vi "Excel_Get_Range.vi"(0 "Excel._Worksheet":refnum<k7>, 5 "start":cluster{"row":i32, "column":i32}={"row"=-1, "column"=-1}, 7 "end":cluster{"row":i32, "column":i32}={"row"=-1, "column"=-1}, 9 "name":string, 11 "error in (no error)":errorcluster) -> (4 "Range":refnum<k7>, 15 "error out":errorcluster)   [LabVIEW 2020, in "NI_ReportGenerationToolkit.lvlib"]
uses:
  <vilib>/addons/_office/NI_ReportGenerationToolkit.lvlib
  <vilib>/Utility/NIReport.llb/NI_ReportGenerationCore.lvlib
panel:
  in  "Excel.Range":refnum<k7>
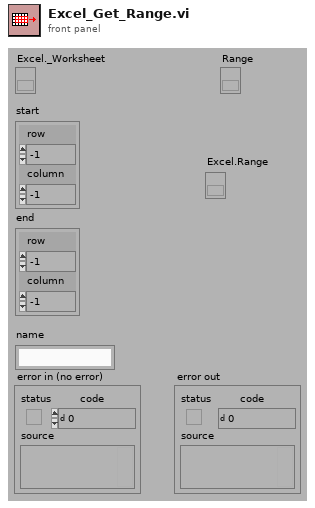
[diagram p1: front panel]
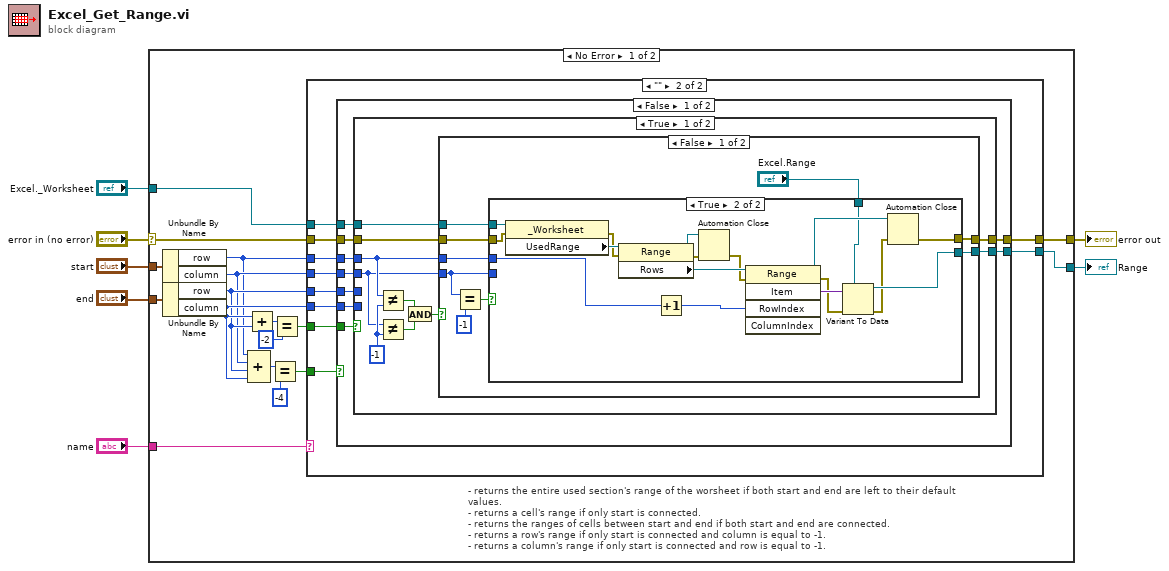
[diagram p0: block diagram]
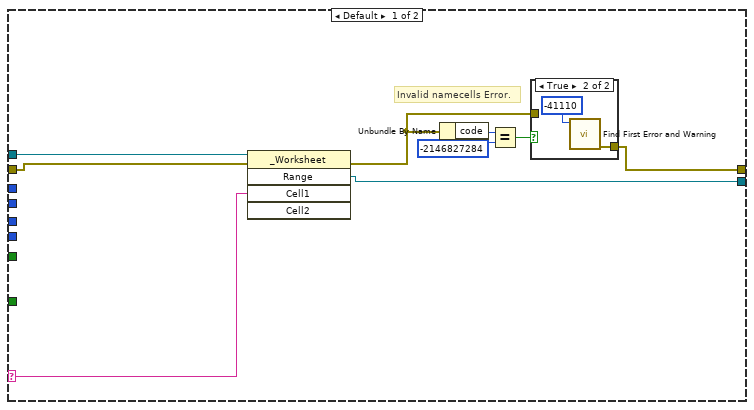
[diagram p2: hidden frame]
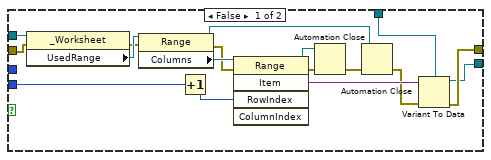
[diagram p4: hidden frame]
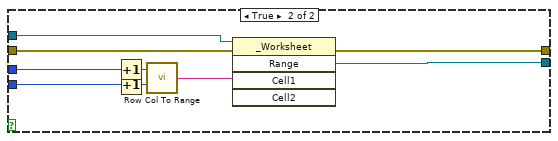
[diagram p5: hidden frame]
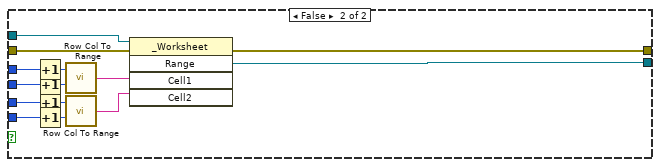
[diagram p6: hidden frame]
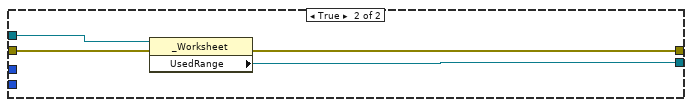
[diagram p7: hidden frame]
diagram:
  n1 = case shown="No Error" "error in (no error)" {
    selector: "error in (no error)" -> [w8 w136]
    tunnel: [w24 _] -> w7
    tunnel: "end" -> [w13 _]
    tunnel: "start" -> [w12 _]
    tunnel: "Excel._Worksheet" -> [w11 _]
    tunnel: [w10 w136] -> w3
    tunnel: "name" -> [w9 _]
    frame No Error {
      # "- returns the entire used section's range of the worsheet if both start and end are left to their default values.\n- returns a cell's range if only start is connected.\n- returns the ranges of cells between start and end if both start and end are connected.\n- returns a row's range if only start is connected and column is equal to -1.\n- returns a column's range if only start is connected and row is equal to -1."
      n2 = Unbundle By Name(w12) -> ("row"=w18:i32, "column"=w19:i32)
      n3 = Unbundle By Name(w13) -> ("row"=w20:i32, "column"=w21:i32)
      n4 = Add(x=w21, y=w20) -> (x+y=w17:i32)
      n5 = Compound Arithmetic op=ADD(w18, w19, w20, w21) -> (w14:i32)
      n6 = Equal?(x=w14, y=-4) -> (x = y?=w23:bool)
      n7 = Equal?(x=w17, y=-2) -> (x = y?=w22:bool)
      n8 = case shown="\"\"" w9 {
        selector: w9 -> [w25 _]
        tunnel: [w31 w46] -> w24
        tunnel: w8 -> [w32 w45]
        tunnel: w23 -> [_ w44]
        tunnel: w22 -> [_ w43]
        tunnel: w21 -> [_ w42]
        tunnel: w20 -> [_ w41]
        tunnel: w19 -> [_ w40]
        tunnel: w18 -> [_ w39]
        tunnel: w11 -> [w33 w38]
        tunnel: [w26 w37] -> w10
        frame Default {
          # "Invalid namecells Error."
          n9 = invoke on="Invoke Node" class="_Worksheet" method="Range"(reference=w33, error in=w32, "Cell1"=w25) -> (error out=w27:errorcluster, "Range"=w31:refnum<k7>)  [unwired: 2 in, 3 out]
          n10 = Unbundle By Name(w27) -> ("code"=w29:i32)
          n11 = Equal?(x=w29, y=-2146827284) -> (x = y?=w30:bool)
          n12 = case shown="True" w30 {
            tunnel: [w34 w35] -> w26
            tunnel: w27 -> [w34 _]
            frame False {
            }
            frame True {
              n13 = call <vilib>:"Find First Error and Warning.vi"("error code"=-41110) -> ("error out"=w35:errorcluster)  [unwired: 1 in, 5 out]
            }
          }
        }
        frame "" {
          n14 = case shown="False" w44 {
            tunnel: w38 -> [w54 w133]
            tunnel: w45 -> [w51 w132]
            tunnel: [w49 w135] -> w46
            tunnel: [w50 w134] -> w37
            tunnel: w43 -> [w55 _]
            tunnel: w39 -> [w53 _]
            tunnel: w40 -> [w52 _]
            tunnel: w41 -> [w48 _]
            tunnel: w42 -> [w47 _]
            frame False {
              n15 = case shown="True" w55 {
                tunnel: w54 -> [w65 w131]
                tunnel: w53 -> [w60 w130]
                tunnel: w52 -> [w59 w129]
                tunnel: w51 -> [w64 w125]
                tunnel: [w63 w124] -> w50
                tunnel: [w62 w123] -> w49
                tunnel: w48 -> [_ w120]
                tunnel: w47 -> [_ w119]
                frame True {
                  w61 = -1
                  n16 = Not Equal?(x=w60, y=w61) -> (x != y?=w57:bool)
                  n17 = Not Equal?(x=w59, y=w61) -> (x != y?=w56:bool)
                  n18 = And(x=w57, y=w56) -> (x .and. y?=w58:bool)
                  n19 = case shown="False" w58 {
                    tunnel: w65 -> [w70 w117]
                    tunnel: w60 -> [w74 w116]
                    tunnel: w59 -> [w73 w115]
                    tunnel: w64 -> [w69 w112]
                    tunnel: [w67 w111] -> w63
                    tunnel: [w68 w110] -> w62
                    frame False {
                      n20 = Equal?(x=w73, y=-1) -> (x = y?=w71:bool)
                      n21 = case shown="True" w71 {
                        tunnel: w73 -> [w90 _]
                        tunnel: w74 -> [_ w107]
                        tunnel: w70 -> [w82 w99]
                        tunnel: w69 -> [w80 w98]
                        tunnel: "Excel.Range" -> [w75 w92]
                        tunnel: [w84 w104] -> w68
                        tunnel: [w85 w102] -> w67
                        frame False {
                          n22 = property on="Property Node" class="_Worksheet"(reference=w82, error in=w80) -> (error out=w79:errorcluster, "UsedRange"=w81:refnum<k7>)  [unwired: 1 out]
                          n23 = property on="Property Node" class="Range"(reference=w81, error in=w79) -> (reference out=w76:refnum<k7>, error out=w87:errorcluster, "Columns"=w91:refnum<k7>)
                          n24 = Increment(x=w90) -> (x+1=w89:i32)
                          n25 = invoke on="Invoke Node" class="Range" method="Item"(reference=w91, error in=w87, "RowIndex"=w89) -> (reference out=w83:refnum<k7>, error out=w88:errorcluster, "Item"=w86:variant)  [unwired: 2 in, 2 out]
                          n26 = Automation Close(3:w88, 5:w83) -> (0:w78:errorcluster)
                          n27 = Automation Close(3:w78, 5:w76) -> (0:w77:errorcluster)
                          n28 = Variant To Data(error in=w77, type=w75, Variant=w86) -> (data=w84:refnum<k7>, error out=w85:errorcluster)
                        }
                        frame True {
                          n29 = property on="Property Node" class="_Worksheet"(reference=w99, error in=w98) -> (error out=w96:errorcluster, "UsedRange"=w97:refnum<k7>)  [unwired: 1 out]
                          n30 = property on="Property Node" class="Range"(reference=w97, error in=w96) -> (reference out=w94:refnum<k7>, error out=w95:errorcluster, "Rows"=w108:refnum<k7>)
                          n31 = Increment(x=w107) -> (x+1=w100:i32)
                          n32 = Automation Close(3:w95, 5:w94) -> (0:w93:errorcluster)
                          n33 = invoke on="Invoke Node" class="Range" method="Item"(reference=w108, error in=w93, "RowIndex"=w100) -> (reference out=w101:refnum<k7>, error out=w105:errorcluster, "Item"=w106:variant)  [unwired: 2 in, 2 out]
                          n34 = Variant To Data(error in=w105, type=w92, Variant=w106) -> (data=w104:refnum<k7>, error out=w103:errorcluster)
                          n35 = Automation Close(3:w103, 5:w101) -> (0:w102:errorcluster)
                        }
                      }
                    }
                    frame True {
                      n36 = Increment(x=w116) -> (x+1=w114:i32)
                      n37 = Increment(x=w115) -> (x+1=w113:i32)
                      n38 = call <vilib>:"Row Col To Range.vi"("Column"=w113, "Row"=w114) -> ("Output String"=w109:string)
                      n39 = invoke on="Invoke Node" class="_Worksheet" method="Range"(reference=w117, error in=w112, "Cell1"=w109) -> (error out=w111:errorcluster, "Range"=w110:refnum<k7>)  [unwired: 2 in, 3 out]
                    }
                  }
                }
                frame False {
                  n40 = Increment(x=w130) -> (x+1=w128:i32)
                  n41 = Increment(x=w129) -> (x+1=w127:i32)
                  n42 = Increment(x=w120) -> (x+1=w121:i32)
                  n43 = Increment(x=w119) -> (x+1=w122:i32)
                  n44 = call <vilib>:"Row Col To Range.vi"("Column"=w127, "Row"=w128) -> ("Output String"=w126:string)
                  n45 = call <vilib>:"Row Col To Range.vi"("Column"=w122, "Row"=w121) -> ("Output String"=w118:string)
                  n46 = invoke on="Invoke Node" class="_Worksheet" method="Range"(reference=w131, error in=w125, "Cell1"=w126, "Cell2"=w118) -> (error out=w124:errorcluster, "Range"=w123:refnum<k7>)  [unwired: 1 in, 3 out]
                }
              }
            }
            frame True {
              n47 = property on="Property Node" class="_Worksheet"(reference=w133, error in=w132) -> (error out=w134:errorcluster, "UsedRange"=w135:refnum<k7>)  [unwired: 1 out]
            }
          }
        }
      }
    }
    frame Error {
    }
  }
  "Range" <- w7
  "error out" <- w3
